vi "Get_Config_Data.vi"(8 "error in (no error)":errorcluster, 11 "Logger_Data In":T1={"Data_Base_Path"=path "", "Log_File_Ref"=refnum, "Timer_Flag"=FALSE, "Log_Interval"=1.0, "Config_Base_Path"=path ""}) -> (0 "error out":errorcluster, 3 "Logger_Data Out":T1={"Data_Base_Path"=path "", "Log_File_Ref"=refnum, "Timer_Flag"=FALSE, "Log_Interval"=1.0, "Config_Base_Path"=path ""})   [LabVIEW 2019, in "Data_Logger.lvlib"]
uses:
  Data_Logger.lvlib
  Logger_Data.ctl
  <vilib>/Utility/config.llb/Read Key (Double).vi
  <vilib>/Utility/config.llb/NI_LVConfig.lvlib
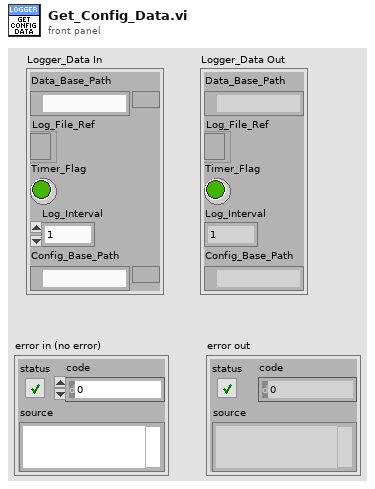
[diagram p1: front panel]
types:
  T1 = typedef "Data_Logger.lvlib/Logger_Data.ctl" = cluster{"Data_Base_Path":path, "Log_File_Ref":refnum<file>, "Timer_Flag":bool, "Log_Interval":dbl, "Config_Base_Path":path}
  T2 = typedef "NI_LVConfig.lvlib/Config Data RefNum.ctl" = refnum<k1>
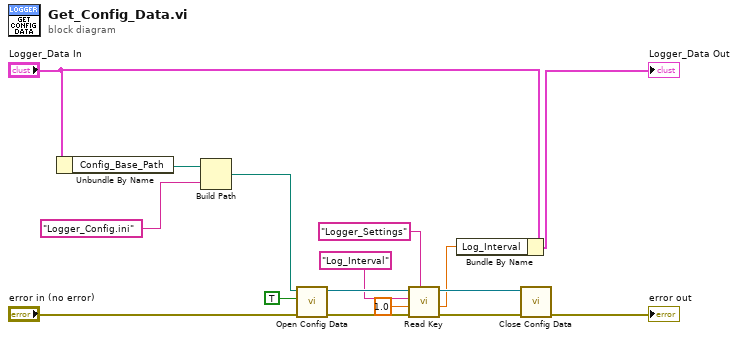
[diagram p0: block diagram]
diagram:
  n1 = Unbundle By Name("Logger_Data In") -> ("Config_Base_Path"=w16:path)
  n2 = Build Path(base path=w16, name or relative path="Logger_Config.ini") -> (appended path=w15:path)
  n3 = call <vilib>:"Open Config Data.vi"("error in (no error)"="error in (no error)", "create file if necessary (T)"=TRUE, "configuration file path"=w15) -> ("error out"=w13:errorcluster, "refnum"=w12:T2)  [unwired: 6 in, 1 out]
  n4 = call-poly <vilib>:"Read Key.vi"("section"="Logger_Settings", "error in (no error)"=w13, "default value"=1.0, "key"="Log_Interval", "refnum"=w12) -> ("error out"=w10:errorcluster, "value"=w1:dbl, "refnum out"=w11:T2)  [unwired: 3 in, 1 out]
  n5 = Bundle By Name(cluster="Logger_Data In", "Log_Interval"=w1) -> (→"Logger_Data Out":T1)
  n6 = call <vilib>:"Close Config Data.vi"("error in (no error)"=w10, "refnum"=w11) -> ("error out"=→"error out":errorcluster)  [unwired: 8 in, 1 out]
